vi "Move Arm.vi"(0 "Target Voltage":dbl) -> ()   [LabVIEW 2015]
panel:
  in  "Speed":dbl=0.35
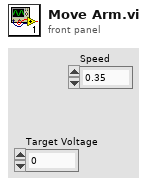
[diagram p1: front panel]
types:
  T1 = typedef "WPI_AnalogChannelDevRef.ctl" = cluster{"DevStatus":errorcluster, "Analog Channel":T2}
  T2 = typedef "FPGA_AIChannel.ctl" = enum8{"AI 0", "AI 1", "AI 2", "AI 3", "AI MXP 0", "AI MXP 1", "AI MXP 2", "AI MXP 3", "Invalid"}
  T3 = typedef "WPI_MotorControlDeviceRef.ctl" = cluster{"DeviceStatus":errorcluster, "Type":T4, "PWM":cluster{"PWM Channel":T5, "DeadBand":T6}, "CAN":cluster{"Device Number":u8, "Control Mode":T7, "Semaphore":T8, "Max Vout":dbl, "TalonSRX Control Mode":T9}, "Invert":bool}
  T4 = typedef "WPI_MotorControlType.ctl" = enum16{"PWM", "CAN", "CANTalonSRX"}
  T5 = typedef "FPGA_DIOPWMChannel.ctl" = enum8{"PWM 0", "PWM 1", "PWM 2", "PWM 3", "PWM 4", "PWM 5", "PWM 6", "PWM 7", "PWM 8", "PWM 9", "PWM MXP 0", "PWM MXP 1", "PWM MXP 2", "PWM MXP 3", "PWM MXP 4", "PWM MXP 5", "PWM MXP 6", "PWM MXP 7", "PWM MXP 8", "PWM MXP 9", "Invalid"}
  T6 = typedef "WPI_PWMDeadband.ctl" = cluster{"Name":string, "maxPositivePwm":i32, "minPositivePwm":i32, "centerPwm":i32, "maxNegativePwm":i32, "minNegativePwm":i32, "angularRange":u16}
  T7 = typedef "WPI_CANJaguar_ControlMode.ctl" = enum8{"Percent VBus", "Current", "Speed", "Position", "Voltage"}
  T8 = typedef "Semaphore RefNum" = refnum<k1>
  T9 = typedef "WPI_CANTalonSRX_APIControlMode.ctl" = enum8{"Percent VBus", "Speed", "Position", "Slave", "Unchanged / Invalid", "Voltage Compensation", "Current", "Motion Profile"}
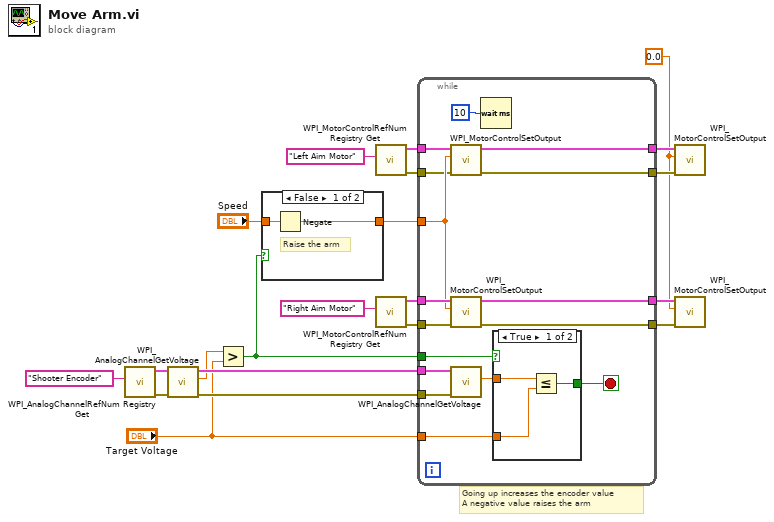
[diagram p0: block diagram]
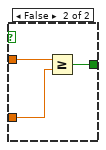
[diagram p3: hidden frame]
diagram:
  w1 = 0.0
  # "Going up increases the encoder value\nA negative value raises the arm"
  n1 = call <vilib>:"WPI_AnalogChannelRefNum Registry Get.vi"("refnum name"="Shooter Encoder") -> ("error out"=w14:errorcluster, "AIDeviceRef"=w16:T1)  [unwired: 9 in]
  n2 = call <vilib>:"WPI_AnalogChannelGetVoltage.vi"("error in (no error)"=w14, "AIDeviceRef"=w16) -> ("error out"=w13:errorcluster, "Voltage"=w11:dbl, "AIDeviceRef"=w15:T1)  [unwired: 7 in]
  n3 = Greater?(x=w11, y="Target Voltage") -> (0:w10:bool)
  n4 = case shown="False" w10 {
    tunnel: "Speed" -> [w23 w24]
    tunnel: [w22 w24] -> w8
    frame False {
      # "Raise the arm"
      n5 = Negate(x=w23) -> (-x=w22:dbl)
    }
    frame True {
      # "Lower the arm"
    }
  }
  n6 = call <vilib>:"WPI_MotorControlRefNum Registry Get.vi"("refnum name"="Left Aim Motor") -> ("error out"=w4:errorcluster, "MotorControlDevRef"=w17:T3)  [unwired: 9 in]
  n7 = call <vilib>:"WPI_MotorControlRefNum Registry Get.vi"("refnum name"="Right Aim Motor") -> ("error out"=w3:errorcluster, "MotorControlDevRef"=w19:T3)  [unwired: 9 in]
  n8 = while {
    tunnel: "Target Voltage" -> [w40]
    tunnel: w15 -> [w38]
    tunnel: w19 -> [w37]
    tunnel: w17 -> [w36]
    tunnel: w10 -> [w34]
    tunnel: w13 -> [w35]
    tunnel: w8 -> [w32]
    tunnel: [w30] -> w7
    tunnel: [w29] -> w6
    tunnel: [w28] -> w5
    tunnel: w4 -> [w27]
    tunnel: w3 -> [w26]
    tunnel: [w25] -> w2
    stop <- w33 stop-if-true
    n9 = call <vilib>:"WPI_MotorControlSetOutput.vi"("error in (no error)"=w27, "Output"=w32, "MotorControlDevRef"=w36) -> ("error out"=w28:errorcluster, "MotorControlDevRef"=w29:T3)  [unwired: 6 in, 1 out]
    n10 = call <vilib>:"WPI_MotorControlSetOutput.vi"("error in (no error)"=w26, "Output"=w32, "MotorControlDevRef"=w37) -> ("error out"=w25:errorcluster, "MotorControlDevRef"=w30:T3)  [unwired: 6 in, 1 out]
    n11 = call <vilib>:"WPI_AnalogChannelGetVoltage.vi"("error in (no error)"=w35, "AIDeviceRef"=w38) -> ("Voltage"=w39:dbl)  [unwired: 7 in, 2 out]
    n12 = Wait (ms)(milliseconds to wait=u32 10) -> ()  [unwired: 1 out]
    n13 = case shown="True" w34 {
      tunnel: w40 -> [w41 w44]
      tunnel: w39 -> [w42 w45]
      tunnel: [w43 w46] -> w33
      frame True {
        n14 = Less Or Equal?(x=w42, y=w41) -> (x <= y?=w43:bool)
      }
      frame False {
        n15 = Greater Or Equal?(x=w45, y=w44) -> (x >= y?=w46:bool)
      }
    }
  }
  n16 = call <vilib>:"WPI_MotorControlSetOutput.vi"("error in (no error)"=w5, "Output"=w1, "MotorControlDevRef"=w6) -> ()  [unwired: 6 in, 3 out]
  n17 = call <vilib>:"WPI_MotorControlSetOutput.vi"("error in (no error)"=w2, "Output"=w1, "MotorControlDevRef"=w7) -> ()  [unwired: 6 in, 3 out]
